vi "ShootTactic.vi"(7 "firstCall?":bool=TRUE, 8 "error in (no error)":errorcluster, 9 "Game in":refnum<class "Game.lvclass">, 10 "Robot":refnum<class "Robot.lvclass">, 11 "ShootTactic in":refnum<class "ShootTactic.lvclass">) -> (0 "error out":errorcluster, 1 "Game out":refnum<class "Game.lvclass">, 2 "Robot out":refnum<class "Robot.lvclass">, 3 "ShootTactic out":refnum<class "ShootTactic.lvclass">)   [LabVIEW 2024, in "ShootTactic.lvclass"]
uses:
  ShootTactic.lvclass
  C:/Users/as119/OneDrive/Documentos/roboIME/SSL_AI/Tactic_class/Tactic.lvclass
  Robot_class/Robot.lvclass
  Game_class/Game.lvclass
  States.ctl
  Robot_class/tactics.ctl
  Tactic_class/Tactic.lvclass/Tactic.ctl
  Game_class/Game.lvclass/Game.ctl
  Events_class/Events.lvclass/Events.ctl
  Parameters_class/Parameters.lvclass/Parameters.ctl
  Robot_class/Robot.lvclass/Robot.ctl
  Object_class/Object.lvclass/Object.ctl
  Ball_class/Ball.lvclass/Ball.ctl
  Skillbook_class/Skillbook.lvclass/Skillbook.ctl
  Field_class/Field.lvclass/Field.ctl
  ShootTactic.lvclass/ShootTactic.ctl
  Game_class/Read BallRef.vi
  Game_class/Read FieldRef.vi
  Game_class/Read Parameters.lvclass.vi
  Parameters_class/Read AttakingOurselves.vi
  Field_class/Read ourGoalPosition.vi
  Field_class/Read enemyGoalPosition.vi
  Object_class/Read x.vi
  Object_class/Read y.vi
  Object_class/Read position(x,y).vi
  Skillbook_class/Read KickToSkill.vi
  Skillbook_class/Read WaitBallTrajSkill.vi
  Parameters_class/Read AttackerFarback.vi
  Skillbook_class/Read AttackerBallInGoalieAreaSkill.vi
  Game_class/Read Utilities.lvclass.vi
  Game_class/Read EventsRef.vi
  Game_class/Read EnemyRef.vi
  Game_class/Read DefensiveTeam.vi
  Game_class/Read NewParameters.vi
  Ball_class/Read velocityNorm.vi
  Events_class/Read ball_inside_enemy_goalie_area.vi
  Events_class/Read ball_inside_our_goalie_area.vi
  Robot_class/Write kick_x.vi
  Robot_class/Write kick_z.vi
  Tactic_class/Read Skillbook.vi
  Write States.vi
  Robot_class/Write tactic.vi
  Robot_class/Read dest_x.vi
  Robot_class/Read dest_y.vi
  Robot_class/Write dest_x.vi
  Robot_class/Write dest_y.vi
  <vilib>/Analysis/_algsub.llb/Vector Norm.vi
  <vilib>/Analysis/_algsub.llb/Real Vector Norm.vi
  Ball_class/Ball.lvclass
  C:/Users/as119/OneDrive/Documentos/roboIME/SSL_AI/Object_class/Object.lvclass
  Utilities_class/Utilities.lvclass
  Events_class/Events.lvclass
  Enemy_class/Enemy.lvclass
  Ally_class/Ally.lvclass
  Parameters_class/Parameters.lvclass
  Field_class/Field.lvclass
  Skillbook_class/Skillbook.lvclass
  KickToSkill_class/KickToSkill.lvclass
  WaitBallTrajSkill_class/WaitBallTrajSkill.lvclass
  AttackerBallInGoalieAreaSkill_class/AttackerBallInGoalieAreaSkill.lvclass
panel:
  out "x .or. y?":bool
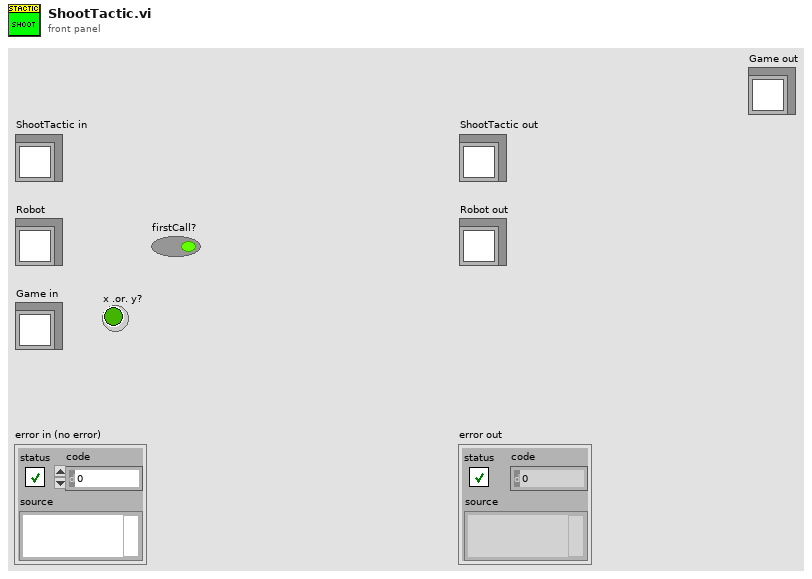
[diagram p1: front panel]
types:
  T1 = typedef "tactics.ctl" = enum16{"GoToBallPlacementPosition", "PlaceBall", "GoToBallPlacement", "5Robots", "BallPlacementEnemy", "ReceivePassInFuturePoint", "Roller", "PrepareRollToPassRollerGoTo", "PrepareRollToPassReceiverGoTo", "WaitRoll", "PositionToRoll", "PenaltyAttacker", "PassObserver", "PenaltyDefense", "TableReceiverTactic", "Test", "DefendGoal", "Marker", "FollowAttacker", "DefendArea", "Shoot", "AttackerAimGoal", "AttackerBallOutOfField", "AttackerBlock", "AttackerStop", "Duelist", "Halt", "ZigZag", "GoTo", "Timeout", "KickToBestRobot", "KickToPassReceiver", "PositionToReceivePass", "WaitPass", "GoToTarget"}
  T2 = typedef "ShootTactic.lvclass/States.ctl" = enum16{"BallInGoalieArea", "Exit", "KickToGoal", "InterceptBall"}
  T3 = typedef "NewParameters.ctl" = cluster{"PenaltyDistance":dbl, "DistanceAttackerToBackBall":dbl, "Division":enum16{"Div B", "Div A"}, "DistanceToAvoidyEnemyRobot":dbl, "BallPlacementDistance":dbl, "DisatanceBehindBallToStealBall":dbl, "MaxDistanceToPositionKickoff":dbl, "BlockEnemyTarget":bool, "MaxStopVAng":dbl, "DistanceMarkerToEnemy":dbl, "IgnoreDribblerContact":bool, "DistanceToBeginEnemyPosession":dbl, "GoToBallWhenEnemyNotMoving":bool, "EnemyDistanceToReduceVelocity":dbl, "TurnOnEnemyDistanceToReduceVelocity":bool, "EnemyDistanceToShootOutBall":dbl, "DefenseKickBall":bool, "MoreKickToGoal? (0-0.3)":dbl, "ChipKickInEnemyField":bool, "ShootOutRobotId":dbl, "FieldLenghtDenominatorInShootOut":dbl, "AdjustPositionInBallPlacement":bool, "PowerGodPass":dbl, "VelocityAbortEnemyPos":dbl, "MaxDistToBeginPass":dbl, "MinDistToBeginPass":dbl, "VelocityInDirects":dbl, "BadDribblerIDs":i32[], "NewKickToDistanceAroundBall":dbl, "PowerAvoidColisionMarker":dbl, "DistanceToAvoidColisionMarker":dbl, "AvoidBallKick":dbl, "DistanceTryKick":dbl, "SuicideKickDIstance":dbl, "AdjustFirstKickDistance":dbl, "AvoidAimLessKick":dbl, "DistanceToAvoidyEnemyShootRobot ":dbl, "NumberOfMarkers":dbl, "PotField":bool, "PIDLateral":bool, "MinDistanceFirstKickX":dbl, "MinDistanceFirstKickY":dbl, "FractionOfDistToTouchGround\nAfterChipKick":dbl, "FractionOfKickxWhen\nComposedWithKickz":dbl, "Style":T4, "MoveInTurnState":bool, "DistFromEnemyToConsider\nMoveInTurnState":dbl, "CascadePID":bool, "TurnAroundParameters":cluster{"Radius":dbl, "Multiplier":dbl, "ChordAngle":dbl}, "SafeDriveVel":dbl, "DistanceToGoToBackBall":dbl, "minDistanceToNotFinish\nEnemyPossession":dbl, "OneTouchShot":cluster{"angleFactor":dbl, "maxAngle":dbl, "Attack":bool, "Defense":bool}, "OpenAngleToGoal":cluster{"minAngle":dbl, "maxAngle":dbl, "minEvaluation":dbl}, "ShotInterception":cluster{"shotSpeed":dbl, "minEnemySpeed":dbl, "maxEnemySpeed":dbl, "minEvaluation":dbl}, "AllyTeamArray":T5[], "maxDefendersNumber":i32, "Zone":cluster{"GuardPositionArray":dbl[][], "ZoneMidField":dbl[], "CenterForwardWidth":dbl}, "MinEvaluationToShoot":dbl, "PassInterception":cluster{"maxPassSpeed":dbl, "minPassSpeed":dbl, "minEnemySpeed":dbl, "chipPassDistance":dbl, "chipPassEvaluation":dbl, "minEvaluation":dbl, "maxEnemySpeed":dbl}, "PassDistance":cluster{"maxDistance":dbl, "minDistance":dbl}, "receiverSpeed":dbl, "maxBallSpeed":dbl, "slackTime":dbl, "Turning radius":dbl, "Turning v_ang":dbl, "AlignError":cluster{"Distance":dbl, "Orientation":dbl, "V_norm(m/s)":dbl, "V_ang (rad/s)":dbl}, "RobotRadius":dbl, "KickerDistance":dbl, "keeper angle  to cover goalpost":dbl, "a_slide":dbl, "a_roll":dbl, "k_switch":dbl, "Penalty":u16}
  T4 = typedef "Style.ctl" = enum16{"Insanity", "Offensive", "Defensive"}
  T5 = typedef "AllyTeam.ctl" = enum16{"Keeper", "Defender", "Attacker"}
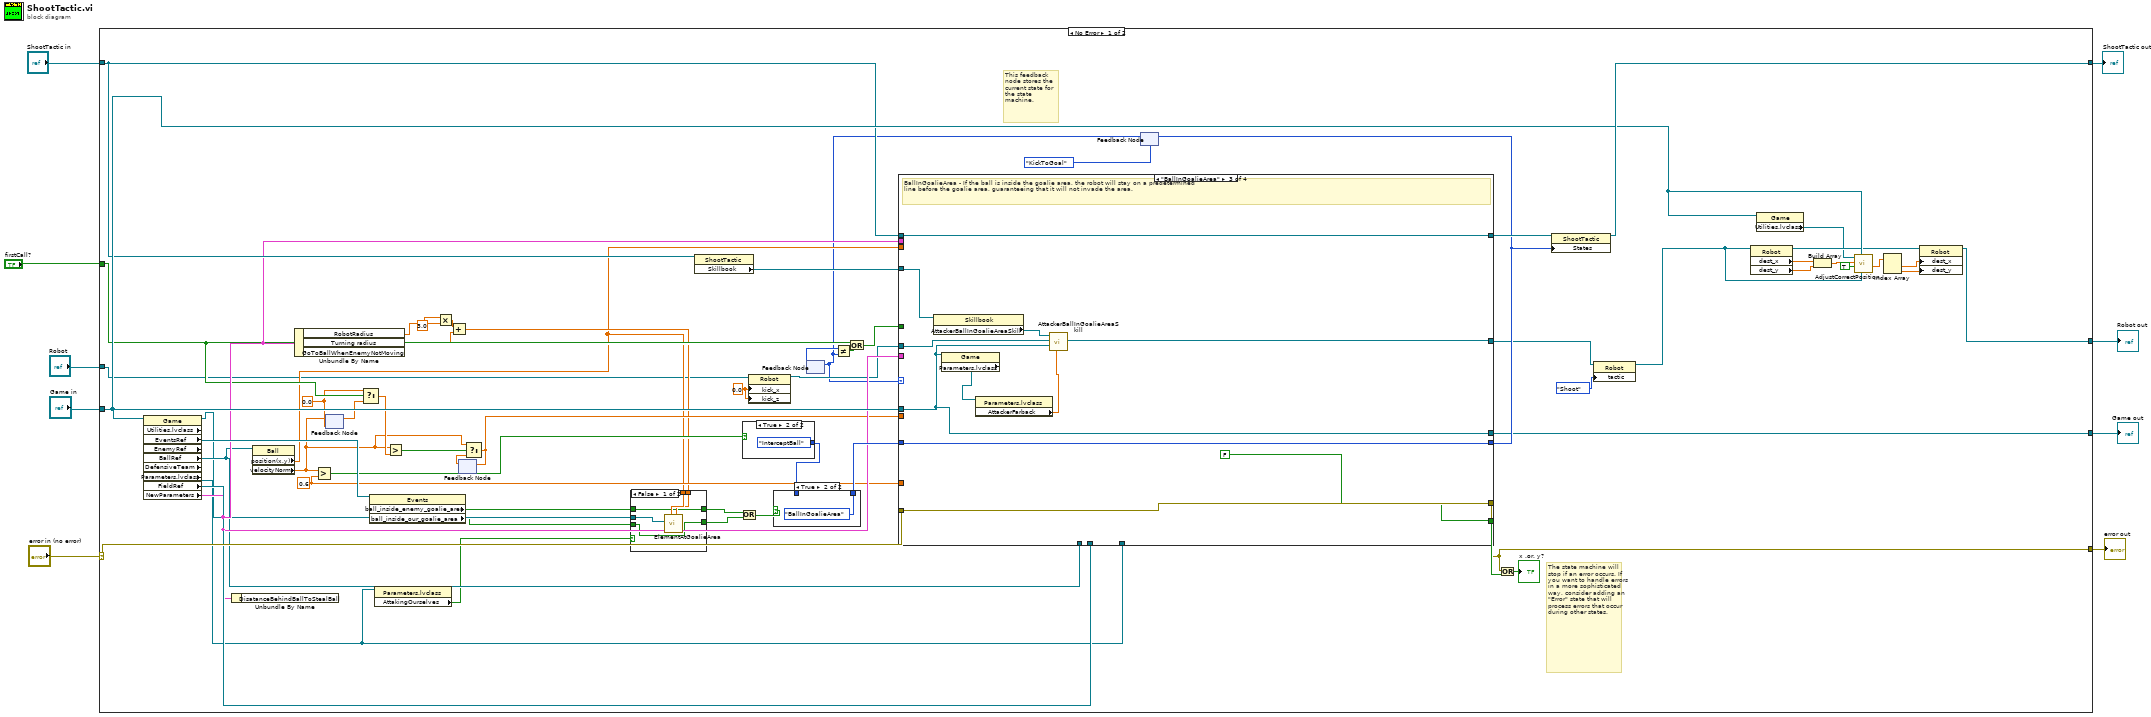
[diagram p0: block diagram]
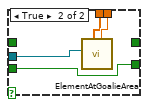
[diagram p2: hidden frame]
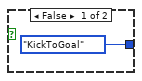
[diagram p4: hidden frame]
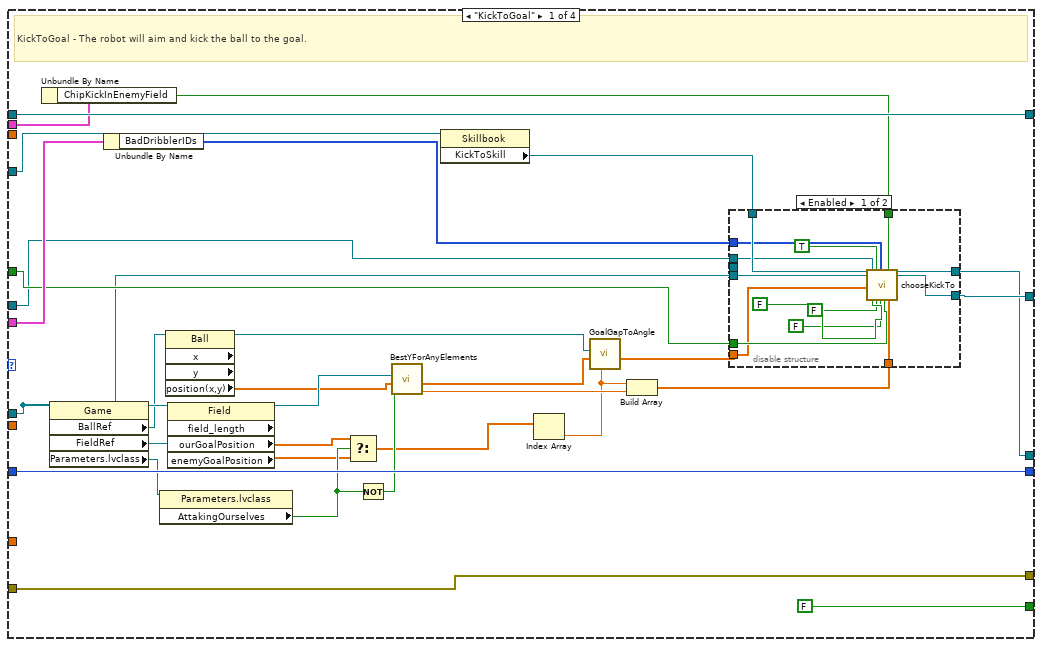
[diagram p5: hidden frame]
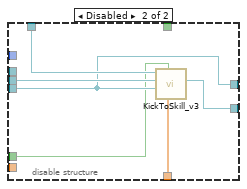
[diagram p6: hidden frame]
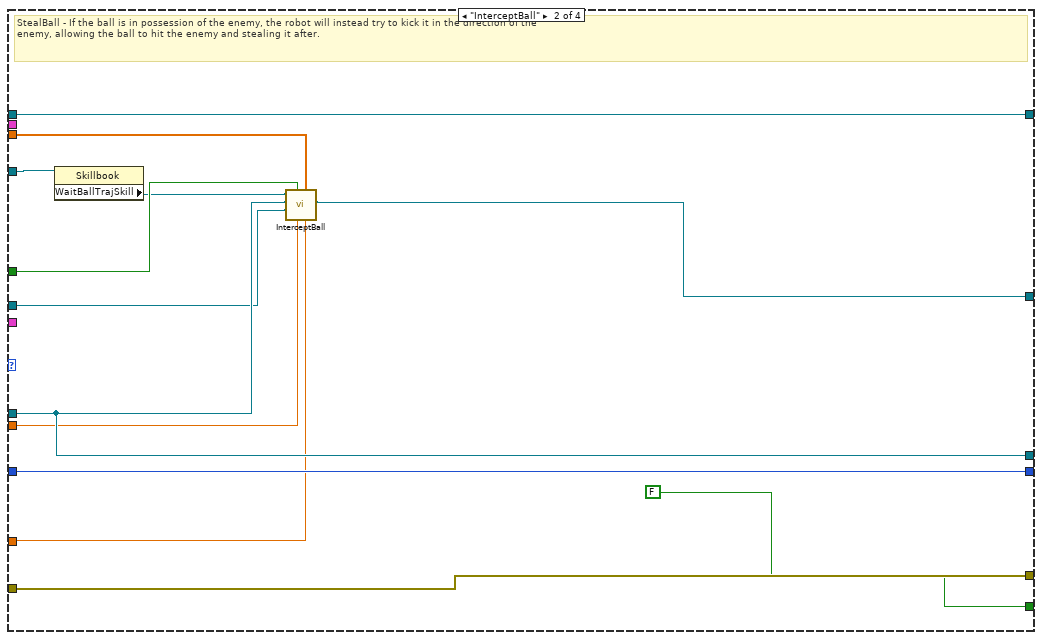
[diagram p7: hidden frame]
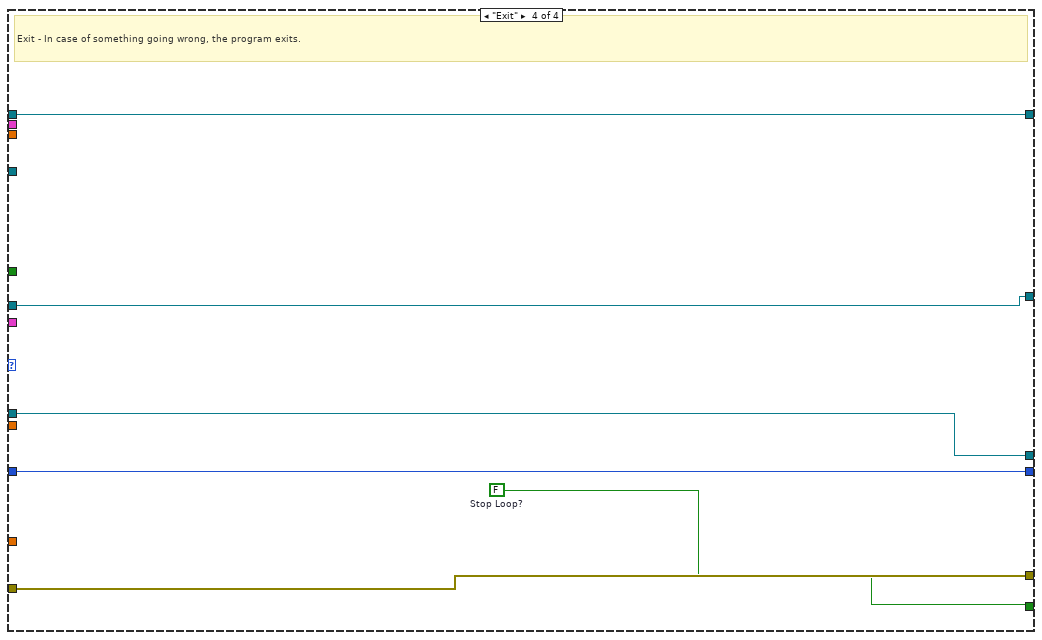
[diagram p8: hidden frame]
diagram:
  n1 = case shown="No Error" "error in (no error)" {
    selector: "error in (no error)" -> [w65 w167]
    tunnel: [w66 w167] -> w8
    tunnel: [w67 w166] -> w6
    tunnel: "ShootTactic in" -> [w50 w166]
    tunnel: "Robot" -> [w12 w165]
    tunnel: "Game in" -> [w56 _]
    tunnel: [w57 w165] -> w3
    tunnel: "firstCall?" -> [w35 _]
    tunnel: [w54 _] -> w1
    frame No Error {
      w13 = 0.0 ("kick_x")
      w32 = 0.0 ("velocityNorm")
      w27 = 0.6 ("y")
      # "The state machine will stop if an error occurs. If you want to handle errors in a more sophisticated way, consider adding an \"Error\" state that will process errors that occur during other states."
      # "This feedback node stores the current state for the state machine."
      n2 = property class="Game" props=["Utilities.lvclass", "EventsRef", "EnemyRef", "BallRef", "DefensiveTeam", "Parameters.lvclass", "FieldRef", "NewParameters"](reference=w56) -> (reference out=w26:refnum<class "Game.lvclass">, "EventsRef"=w58:refnum<class "Events.lvclass">, "BallRef"=w37:refnum<class "Ball.lvclass">, "Parameters.lvclass"=w16:refnum<class "Parameters.lvclass">, "FieldRef"=w40:refnum<class "Field.lvclass">, "NewParameters"=w39:T3)  [unwired: 1 in, 4 out]
      n3 = Unbundle By Name(w39) -> ()  [unwired: 1 out]
      n4 = property class="Ball"(reference=w37) -> ("position(x,y)"=w14:dbl[], "velocityNorm"=w30:dbl)  [unwired: 1 in, 2 out]
      n5 = Unbundle By Name(w39) -> ("RobotRadius"=w22:dbl, "Turning radius"=w24:dbl)  [unwired: 1 out]
      n6 = Greater?(x=w30, y=w27) -> (0:w36:bool)
      n7 = feedback-in #1(w30) -> ()
      n8 = feedback #1(w32) -> (w33:dbl)
      n9 = Select(t=w32, s=w35, f=w33) -> (s? t:f=w34:dbl)
      n10 = property class="Events"(reference=w58) -> ("ball_inside_enemy_goalie_area"=w18:bool, "ball_inside_our_goalie_area"=w17:bool)  [unwired: 1 in, 2 out]
      n11 = property class="Parameters.lvclass"(reference=w16) -> ("AttakingOurselves"=w15:bool)  [unwired: 1 in, 2 out]
      n12 = Greater?(x=w30, y=w34) -> (0:w31:bool)
      n13 = Multiply(x=3.0, y=w22) -> (x*y=w23:dbl)
      n14 = Add(x=w23, y=w24) -> (x+y=w20:dbl)
      n15 = feedback #2() -> (w29:dbl)  [unwired: 1 in]
      n16 = Select(t=w30, s=w31, f=w29) -> (s? t:f=w28:dbl)
      n17 = feedback-in #2(w28) -> ()
      n18 = case shown="False" w15 {
        tunnel: w14 -> [w76 w79]
        tunnel: w26 -> [w75 w78]
        tunnel: [w72 w77] -> w25
        tunnel: w20 -> [w74 w80]
        tunnel: [w73 _] -> w19
        tunnel: w18 -> [w73 _]
        tunnel: w17 -> [w72 w77]
        frame False {
          n19 = call "ElementAtGoalieArea.vi"("ElementRadius"=w74, "Elemento pos."=w76, "Game"=w75) -> ()  [unwired: 4 in, 5 out]
        }
        frame True {
          n20 = call "ElementAtGoalieArea.vi"("ElementRadius"=w80, "Elemento pos."=w79, "Game"=w78) -> ()  [unwired: 4 in, 5 out]
        }
      }
      n21 = property class="ShootTactic"(reference=w50) -> ("Skillbook"=w69:refnum<class "Skillbook.lvclass">)  [unwired: 1 in, 2 out]
      n22 = Or(x=w19, y=w25) -> (x .or. y?=w62:bool)
      n23 = case shown="True" w36 {
        tunnel: [States."KickToGoal" ("States") States."InterceptBall" ("States")] -> w60
        frame False {
        }
        frame True {
        }
      }
      n24 = property class="Robot"(reference=w12, "kick_x"=w13, "kick_z"=w13) -> (reference out=w11:refnum<class "Robot.lvclass">)  [unwired: 1 in, 1 out]
      n25 = case shown="True" w62 {
        tunnel: [w81 States."BallInGoalieArea" ("States")] -> w61
        tunnel: w60 -> [w81 _]
        frame False {
        }
        frame True {
        }
      }
      n26 = feedback #3() -> (w51:T2)  [unwired: 1 in]
      n27 = feedback #4(States."KickToGoal" ("States")) -> (w10:T2)
      n28 = feedback-in #3(w10) -> ()
      n29 = Not Equal?(x=w51, y=w10) -> (x != y?=w52:bool)
      n30 = Or(x=w35, y=w52) -> (x .or. y?=w53:bool)
      n31 = case shown="\"BallInGoalieArea\"" w10 {
        tunnel: [FALSE ("Stop Loop?") FALSE ("Stop Loop?") FALSE ("Stop Loop?") w161] -> w71
        tunnel: w65 -> [w113 w147 w158 w164]
        tunnel: [w113 w147 w158 w164] -> w66
        tunnel: w69 -> [w112 w143 w154 _]
        tunnel: [w107 w139 w152 w159] -> w55
        tunnel: [w111 w144 w157 w163] -> w68
        tunnel: w50 -> [w111 w144 w157 w163]
        tunnel: w56 -> [w98 w140 w149 w160]
        tunnel: w61 -> [w110 w146 w155 w162]
        tunnel: [w110 w146 w155 w162] -> w63
        tunnel: w53 -> [w100 w142 _ _]
        tunnel: [w105 w140 w149 w160] -> w54
        tunnel: w37 -> [_ _ _ _]
        tunnel: w40 -> [_ _ _ _]
        tunnel: w39 -> [w104 _ _ _]
        tunnel: w39 -> [w103 _ _ _]
        tunnel: w16 -> [_ _ _ _]
        tunnel: w11 -> [w85 w136 w148 w159]
        tunnel: w28 -> [_ w138 _ _]
        tunnel: w27 -> [_ w137 _ _]
        tunnel: w14 -> [_ w135 _ _]
        frame "KickToGoal" {
          # "KickToGoal - The robot will aim and kick the ball to the goal."
          n32 = Unbundle By Name(w104) -> ("ChipKickInEnemyField"=w99:bool)
          n33 = property class="Game"(reference=w98) -> ("BallRef"=w97:refnum<class "Ball.lvclass">, "FieldRef"=w109:refnum<class "Field.lvclass">, "Parameters.lvclass"=w108:refnum<class "Parameters.lvclass">)  [unwired: 1 in, 2 out]
          n34 = Unbundle By Name(w103) -> ("BadDribblerIDs"=w101:i32[])
          n35 = property class="Parameters.lvclass"(reference=w108) -> ("AttakingOurselves"=w93:bool)  [unwired: 1 in, 2 out]
          n36 = property class="Ball" props=["x", "y", "position(x,y)"](reference=w97) -> (reference out=w89:refnum<class "Ball.lvclass">, "position(x,y)"=w96:dbl[])  [unwired: 1 in, 3 out]
          n37 = property class="Field" props=["field_length", "ourGoalPosition", "enemyGoalPosition"](reference=w109) -> ("ourGoalPosition"=w92:dbl[], "enemyGoalPosition"=w91:dbl[])  [unwired: 1 in, 3 out]
          n38 = Select(t=w92, s=w93, f=w91) -> (s? t:f=w86:dbl[])
          n39 = Not(x=w93) -> (.not. x?=w94:bool)
          n40 = call "BestYForAnyElements.vi"("inimigos"=w94, "Position to be analyzed"=w96, "Game"=w98) -> ("Best y"=w95:dbl, "Gap Coord"=w88:dbl[])  [unwired: 5 in, 2 out]
          n41 = property class="Skillbook"(reference=w112) -> ("KickToSkill"=w102:refnum<class "KickToSkill.lvclass">)  [unwired: 1 in, 2 out]
          n42 = Index Array(array=w86) -> (element=w87:dbl)  [unwired: 1 in]
          n43 = call "GoalGapToAngle.vi"("x_goal"=w87, "GoalGap"=w88, "Ball"=w89) -> ("angle gap"=w90:dbl[])  [unwired: 6 in, 2 out]
          n44 = Build Array(w87, w95) -> (w106:dbl[])
          n45 = disable-structure shown="Enabled" {
            disable-tunnel: [w128 w131] -> w107
            disable-tunnel: w106 -> [w127 w132]
            disable-tunnel: [w126 w130] -> w105
            disable-tunnel: _ -> [_ w133]
            disable-tunnel: w102 -> [w125 w134]
            disable-tunnel: w98 -> [w124 w130]
            disable-tunnel: w101 -> [w123 _]
            disable-tunnel: w100 -> [w120 w129]
            disable-tunnel: w99 -> [w117 _]
            disable-tunnel: w90 -> [w116 _]
            disable-tunnel: w85 -> [w115 _]
            frame Enabled {
              n46 = call "chooseKickTo.vi"("KickToSkill in"=w125, "Game in"=w124, "target gap"=w116, "Robot"=w115, "KickForce 0?"=FALSE, "use criteria?"=TRUE, "ForceInGame"=FALSE, "BadDribblerIDs"=w123, "pass?"=FALSE, "firstCall"=w120, "ChipKickInEnemyField"=w117, "Target"=w127) -> ("Game out"=w126:refnum<class "Game.lvclass">, "Robot out"=w128:refnum<class "Robot.lvclass">)  [unwired: 14 in]
            }
            frame Disabled {
              n47 = call "KickToSkill_v3.vi"("kick_x"=w132, "firstCall?"=w129, "Game"=w130, "Robot"=w133, "KickToSkill in"=w134) -> ("Robot out"=w131:refnum<class "Robot.lvclass">)  [unwired: 4 in, 2 out]
            }
          }
        }
        frame "InterceptBall" {
          # "StealBall - If the ball is in possession of the enemy, the robot will instead try to kick it in the direction of the \nenemy, allowing the ball to hit the enemy and stealing it after."
          n48 = property class="Skillbook"(reference=w143) -> ("WaitBallTrajSkill"=w141:refnum<class "WaitBallTrajSkill.lvclass">)  [unwired: 1 in, 2 out]
          n49 = call "InterceptBall.vi"("vf"=w137, "target"=w135, "vi"=w138, "firstCall"=w142, "Robot"=w136, "Game"=w140, "WaitBallTrajSkill in"=w141) -> ("robot out"=w139:refnum<class "Robot.lvclass">)  [unwired: 2 in, 2 out]
        }
        frame "BallInGoalieArea" {
          # "BallInGoalieArea - If the ball is inside the goalie area, the robot will stay on a predetermined\nline before the goalie area, guaranteeing that it will not invade the area."
          n50 = property class="Skillbook"(reference=w154) -> ("AttackerBallInGoalieAreaSkill"=w153:refnum<class "AttackerBallInGoalieAreaSkill.lvclass">)  [unwired: 1 in, 2 out]
          n51 = property class="Game"(reference=w149) -> ("Parameters.lvclass"=w151:refnum<class "Parameters.lvclass">)  [unwired: 1 in, 2 out]
          n52 = property class="Parameters.lvclass"(reference=w151) -> ("AttackerFarback"=w150:dbl)  [unwired: 1 in, 2 out]
          n53 = call-dynamic "AttackerBallInGoalieAreaSkill.vi"("AttackerFarback"=w150, "Game"=w149, "Robot"=w148, "AttackerBallInGoalieAreaSkill in"=w153) -> ("Robot out"=w152:refnum<class "Robot.lvclass">)  [unwired: 5 in, 2 out]
        }
        frame "Exit" {
          w161 = FALSE  # Stop Loop?
          # "Exit - In case of something going wrong, the program exits."
        }
      }
      n54 = feedback-in #4(w63) -> ()
      n55 = Or(x=w66, y=w71) -> (x .or. y?=→"x .or. y?":bool)
      n56 = property class="ShootTactic"(reference=w68, "States"=w63) -> (reference out=w67:refnum<class "ShootTactic.lvclass">)  [unwired: 1 in, 1 out]
      n57 = property class="Robot"(reference=w55, "tactic"=tactics."Shoot") -> (reference out=w38:refnum<class "Robot.lvclass">)  [unwired: 1 in, 1 out]
      n58 = property class="Robot"(reference=w38) -> (reference out=w46:refnum<class "Robot.lvclass">, "dest_x"=w49:dbl, "dest_y"=w48:dbl)  [unwired: 1 in, 1 out]
      n59 = property class="Game"(reference=w56) -> ("Utilities.lvclass"=w42:refnum<class "Utilities.lvclass">)  [unwired: 1 in, 2 out]
      n60 = Build Array(w49, w48) -> (w47:dbl[])
      n61 = call "AdjustCorrectPosition.vi"("Robot"=w38, "Game"=w56, "IsShoot?"=TRUE, "Position"=w47, "Utilities in"=w42) -> ("AdjustPosition"=w45:dbl[])  [unwired: 4 in, 2 out]
      n62 = Index Array(array=w45) -> (element #1=w44:dbl, element #2=w43:dbl)  [unwired: 2 in]
      n63 = property class="Robot"(reference=w46, "dest_x"=w44, "dest_y"=w43) -> (reference out=w57:refnum<class "Robot.lvclass">)  [unwired: 1 in, 1 out]
    }
    frame Error {
    }
  }
  "error out" <- w8
  "ShootTactic out" <- w6
  "Robot out" <- w3
  "Game out" <- w1
